vi "闪屏.vi"() -> ()   [LabVIEW 2013]
panel:
  out "滑动杆":u8(slide) scale=0.0..100.0
  # "此处可增加动画闪屏效果"
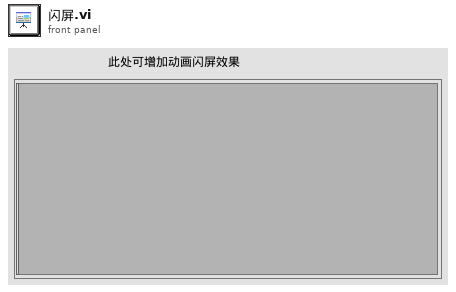
[diagram p1: front panel]
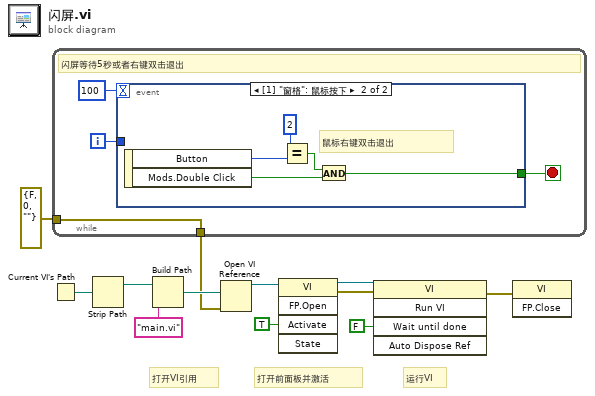
[diagram p0: block diagram]
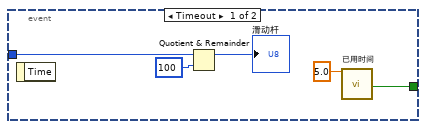
[diagram p2: hidden frame]
diagram:
  # "运行VI"
  # "打开前面板并激活"
  # "打开VI引用"
  n1 = Current VI's Path() -> (path=w11:path)
  n2 = while {
    tunnel: errorcluster {"status"=FALSE, "code"=0, "source"=""} ("错误输入（无错误）") -> [w13]
    tunnel: [w13] -> w2
    i -> [w14]
    stop <- w15 stop-if-true
    # "闪屏等待5秒或者右键双击退出"
    n3 = event shown="[1] \"窗格\": 鼠标按下" {
      selector: _ -> [_ _]
      dyn-events: _ -> [_ _]
      timeout: 100 -> [_ _]
      tunnel: [w20 w22] -> w15
      tunnel: w14 -> [w19 _]
      event Timeout {
        n4 = event-data() -> ()  [unwired: 1 in, 1 out]
        n5 = Quotient & Remainder(x=w19, y=100) -> (x-y*floor(x/y)=→"滑动杆":i32)  [unwired: 1 out]
        n6 = call "已用时间"("Time Target (s)"=5.0) -> ("Time has Elapsed"=w20:bool)  [unwired: 11 in, 7 out]
      }
      event Mouse Down {
        # "鼠标右键双击退出"
        n7 = event-data() -> ("Button"=w26:u16, "Mods.Double Click"=w23:bool)  [unwired: 1 in]
        n8 = Equal?(x=u16 2 ("y"), y=w26) -> (x = y?=w24:bool)
        n9 = And(x=w24, y=w23) -> (x .and. y?=w22:bool)
      }
    }
  }
  n10 = Strip Path(path=w11) -> (stripped path=w10:path)  [unwired: 1 out]
  n11 = Build Path(base path=w10, name or relative path="main.vi" ("名称或相对路径")) -> (appended path=w8:path)
  n12 = Open VI Reference(vi path=w8, error in (no error)=w2) -> (vi reference=w7:refnum<vi>)  [unwired: 4 in, 1 out]
  n13 = invoke class="VI" method="FP.Open"(reference=w7, "Activate"=TRUE ("激活？")) -> (reference out=w5:refnum<vi>, error out=w4:errorcluster)  [unwired: 3 in, 3 out]
  n14 = invoke class="VI" method="Run VI"(reference=w5, error in=w4, "Wait until done"=FALSE ("结束前等待")) -> (error out=w1:errorcluster)  [unwired: 2 in, 4 out]
  n15 = invoke class="VI" method="FP.Close"(error in=w1) -> ()  [unwired: 2 in, 3 out]
